vi "Set Preview Picture Zoom to Fit Image.vi"(8 "error in (no error)":errorcluster, 10 "Size":T2, 11 "UI in":refnum<class "UI.lvclass">) -> (0 "error out":errorcluster, 2 "Offset":T1)   [LabVIEW 2020, in "AR Example.lvlib" / "UI.lvclass"]
uses:
  UI.lvclass
  g_ar_toolkit.common/Image Size (Integer).ctl
  g_ar_toolkit.image/Image Draw Offset.ctl
  UI.lvclass/UI.ctl
  g_ar_toolkit.image/g_ar_toolkit.image.lvlib
  g_ar_toolkit.common/g_ar_toolkit.common.lvlib
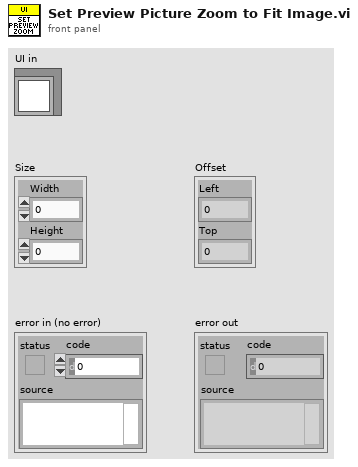
[diagram p1: front panel]
types:
  T1 = typedef "g_ar_toolkit.image.lvlib/Image Draw Offset.ctl" = cluster{"Left":i16, "Top":i16}
  T2 = typedef "g_ar_toolkit.common.lvlib/Image Size (Integer).ctl" = cluster{"Width":u16, "Height":u16}
  T3 = typedef "LVBoundsTypeDef.ctl" = cluster{"Width":u32, "Height":u32}
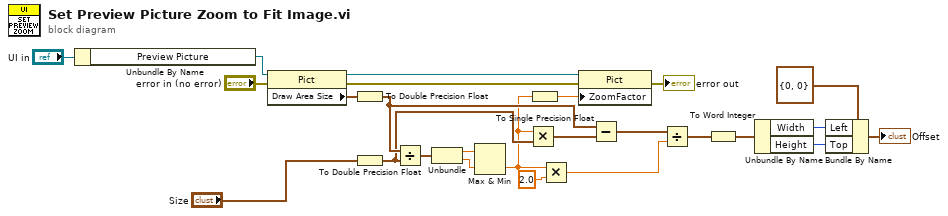
[diagram p0: block diagram]
diagram:
  n1 = Unbundle By Name("UI in") -> ("Preview Picture"=w24:refnum<vi>)
  n2 = property class="Pict"(reference=w24, error in="error in (no error)") -> (reference out=w19:refnum<vi>, error out=w18:errorcluster, "Draw Area Size"=w13:T3)
  n3 = To Double Precision Float(number=w13) -> (double precision float=w11:cluster{"Width":dbl, "Height":dbl})
  n4 = To Double Precision Float(number="Size") -> (double precision float=w10:cluster{"Width":dbl, "Height":dbl})
  n5 = Divide(x=w11, y=w10) -> (x/y=w22:cluster{"Width":dbl, "Height":dbl})
  n6 = Unbundle(w22) -> ("Width"=w20:dbl, "Height"=w21:dbl)
  n7 = Max & Min(x=w20, y=w21) -> (min(x,y)=w1:dbl)  [unwired: 1 out]
  n8 = Multiply(x=w1, y=w10) -> (x*y=w14:cluster{"Width":dbl, "Height":dbl})
  n9 = To Single Precision Float(number=w1) -> (single precision float=w15:sgl)
  n10 = Multiply(x=w1, y=2.0) -> (x*y=w2:dbl)
  n11 = property class="Pict"(reference=w19, error in=w18, "ZoomFactor"=w15) -> (error out=→"error out":errorcluster)  [unwired: 1 out]
  n12 = Subtract(x=w11, y=w14) -> (x-y=w12:cluster{"Width":dbl, "Height":dbl})
  n13 = Divide(x=w12, y=w2) -> (x/y=w8:cluster{"Width":dbl, "Height":dbl})
  n14 = To Word Integer(number=w8) -> (16bit integer=w6:cluster{"Width":i16, "Height":i16})
  n15 = Unbundle By Name(w6) -> ("Width"=w5:i16, "Height"=w4:i16)
  n16 = Bundle By Name(cluster=T1 {"Left"=0, "Top"=0} ("Image Draw Offset"), "Left"=w5, "Top"=w4) -> (→"Offset":T1)
